vi "Read.vi"(7 "Enable Sound":bool, 8 "error in (no error)":errorcluster, 9 "Audio Channels":cluster{"Left":i32, "Right":i32}, 11 "Electrophysiology in":refnum<class "Electrophysiology.lvclass">) -> (0 "error out":errorcluster, 2 "Samples":u32, 3 "Electrophysiology out":refnum<class "Electrophysiology.lvclass">)   [LabVIEW 2014, in "Electrophysiology.lvclass"]
uses:
  Electrophysiology.lvclass
  Electrophysiology.lvclass/Electrophysiology.ctl
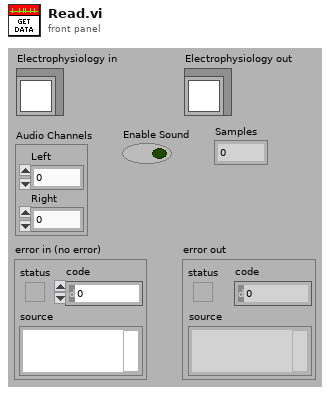
[diagram p1: front panel]
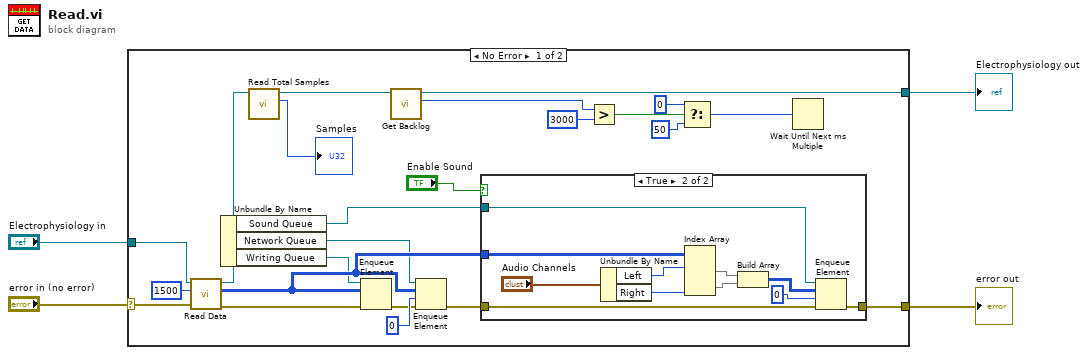
[diagram p0: block diagram]
diagram:
  n1 = case shown="No Error" "error in (no error)" {
    selector: "error in (no error)" -> [w25 w41]
    tunnel: [w27 w41] -> w3
    tunnel: [w6 w40] -> w1
    tunnel: "Electrophysiology in" -> [w26 w40]
    frame No Error {
      n2 = call-dynamic "Read Data.vi"("error in (no error)"=w25, "Read Size"=1500, "AcquireTraces in"=w26) -> ("error out"=w24:errorcluster, "data"=w21:i32[][], "AcquireTraces out"=w23:refnum<class "Electrophysiology.lvclass">)  [unwired: 6 in]
      n3 = Unbundle By Name(w23) -> ("Sound Queue"=w15:refnum<queue>, "Network Queue"=w19:refnum<queue>, "Writing Queue"=w18:refnum<queue>)
      n4 = call-dynamic "Read Total Samples.vi"("AcquireTraces in"=w23) -> ("Total Samples"=→"Samples":u64, "AcquireTraces out"=w7:refnum<class "Electrophysiology.lvclass">)  [unwired: 8 in, 1 out]
      n5 = Enqueue Element(queue=w18, element=w21, error in (no error)=w24) -> (error out=w17:errorcluster)  [unwired: 1 in, 2 out]
      n6 = call-dynamic "Get Backlog.vi"("AcquireTraces in"=w7) -> ("Backlog"=w5:u32, "AcquireTraces out"=w6:refnum<class "Electrophysiology.lvclass">)  [unwired: 8 in, 1 out]
      n7 = Enqueue Element(queue=w19, element=w21, timeout in ms (-1)=0, error in (no error)=w17) -> (error out=w16:errorcluster)  [unwired: 2 out]
      n8 = case shown="True" "Enable Sound" {
        tunnel: w15 -> [_ w37]
        tunnel: w16 -> [w28 w36]
        tunnel: [w28 w34] -> w27
        tunnel: w21 -> [_ w33]
        frame False {
        }
        frame True {
          n9 = Unbundle By Name("Audio Channels") -> ("Left"=w39:i32, "Right"=w30:i32)
          n10 = Index Array(array=w33, index (row) #1=w39, index (row) #2=w30) -> (element #1=w31:i32[], element #2=w29:i32[])  [unwired: 2 in]
          n11 = Build Array(w31, w29) -> (w32:i32[][])
          n12 = Enqueue Element(queue=w37, element=w32, timeout in ms (-1)=0, error in (no error)=w36) -> (error out=w34:errorcluster)  [unwired: 2 out]
        }
      }
      n13 = Greater?(x=w5, y=u32 3000) -> (0:w11:bool)
      n14 = Select(t=0, s=w11, f=u32 50 ("millisecond multiple")) -> (s? t:f=w8:u32)
      n15 = Wait Until Next ms Multiple(millisecond multiple=w8) -> ()  [unwired: 1 out]
    }
    frame Error {
    }
  }
  "error out" <- w3
  "Electrophysiology out" <- w1
